vi "InitializeFpgaAcquisition.vi"(8 "error in (no error)":errorcluster, 11 "923x Acquisition Config":T1={"Acq"=FALSE, "NumberOfModules"=0, "Dynamic FPGA VI Ref"=refnum, "KeyphasorX3"=[], "FixedSizeX32"={"EnabledChannels"=[], "Sensitivity"=[], "InputConfig"=[]}, "SamplingInfo"={"Number of Channels"=4, "Sampling Rate"=4.0, "Channels"=[], "Units"=[], "Offsets"=[]}, "Normal Mode Sample Rate"=0.0, "BlockSize (sec)"=0.0, "Samples To Read (per chan)"=0, "RunningAcquisitionLength"=0.0, "Settling Time"=0.0, "Waveform Groups"=[], "Acquisition Block Number"=0, "Device Name"="", "ValidConfig"=FALSE, "Last Dynamic Module"="", "HighPassFilterState"=[], "Low Frequency Cutoff"=[], "BurstMode"={"Acquisition Time"=0.0, "Sample Rate"=0.0}} {"HighPassFilterState"."Filter State" format="%.2f"; "HighPassFilterState"."IIR Filter Cluster"."Forward Coefficients" format="%.2f"; "HighPassFilterState"."IIR Filter Cluster"."Reverse Coefficients" format="%.2f"; "FixedSizeX32"."InputConfig" items=["AC Coupled", "DC Coupled", "IEPE AC Coupled"]}) -> (0 "error out":errorcluster, 1 "start acquisition?":bool, 2 "dynamic FPGA VI reference":refnum<k20>, 3 "923x Acquisition Config out":T1={"Acq"=FALSE, "NumberOfModules"=0, "Dynamic FPGA VI Ref"=refnum, "KeyphasorX3"=[], "FixedSizeX32"={"EnabledChannels"=[], "Sensitivity"=[], "InputConfig"=[]}, "SamplingInfo"={"Number of Channels"=4, "Sampling Rate"=4.0, "Channels"=[], "Units"=[], "Offsets"=[]}, "Normal Mode Sample Rate"=0.0, "BlockSize (sec)"=0.0, "Samples To Read (per chan)"=0, "RunningAcquisitionLength"=0.0, "Settling Time"=0.0, "Waveform Groups"=[], "Acquisition Block Number"=0, "Device Name"="", "ValidConfig"=FALSE, "Last Dynamic Module"="", "HighPassFilterState"=[], "Low Frequency Cutoff"=[], "BurstMode"={"Acquisition Time"=0.0, "Sample Rate"=0.0}} {"HighPassFilterState"."Filter State" format="%.2f"; "HighPassFilterState"."IIR Filter Cluster"."Forward Coefficients" format="%.2f"; "HighPassFilterState"."IIR Filter Cluster"."Reverse Coefficients" format="%.2f"; "FixedSizeX32"."InputConfig" items=["AC Coupled", "DC Coupled", "IEPE AC Coupled"]})   [LabVIEW 2017, in "CmsAcquisition.lvlib"]
doc: "Initializes the acquisition of the dynamic channels with the RIO Wfm API."
uses:
  <vilib>/addons/InsightCM/Devices/Shared/Cms/CmsAcquisition/CmsAcquisition.lvlib
  <vilib>/addons/InsightCM/Devices/Shared/Cms/CmsAcquisition/controls/Configuration.ctl
  <vilib>/addons/InsightCM/Devices/Shared/Cms/CmsAcquisition/controls/TachometerConfig.ctl
  <vilib>/addons/InsightCM/Devices/Shared/Cms/CmsAcquisition/controls/FixedSizeArrays.ctl
  <vilib>/LabVIEW Targets/FPGA/cRIO/shared/nicrio_ModuleControls/nicrio_cRIO-9232_ConfigModeRing.ctl
  <vilib>/addons/InsightCM/Devices/Shared/Cms/cRIOWfmAcq/subVIs/RIO Wfm Cust Ctrls/rwfm_SamplingInfo.ctl
  <vilib>/addons/InsightCM/Devices/Shared/Cms/CmsAcquisition/controls/Group.ctl
  <vilib>/addons/InsightCM/Devices/Shared/Cms/CmsAcquisition/controls/Channel.ctl
  <vilib>/addons/InsightCM/Utilities/Analysis/Vibration/controls/HighPassFilterState.ctl
  <vilib>/addons/InsightCM/Devices/Shared/Cms/CmsAcquisition/controls/BurstMode.ctl
  <vilib>/Utility/error.llb/Error Cluster From Error Code.vi
  <vilib>/rvi/errors/niLvFpgaAdjustHostInterfaceError.vi
  <vilib>/rvi/interface/nirviReadWriteControl/nirviReadWriteControl.xnode
  <vilib>/addons/InsightCM/Devices/Shared/Cms/cRIOWfmAcq/cRIOWfmLib.lvlib
  NiFpgaLv.dll
  <vilib>/rvi/interface/Simulation/niFpgaSimulationCallBeginRW.vi
  <vilib>/addons/InsightCM/Utilities/Analysis/Vibration/VibrationAnalysisFunctions.lvlib
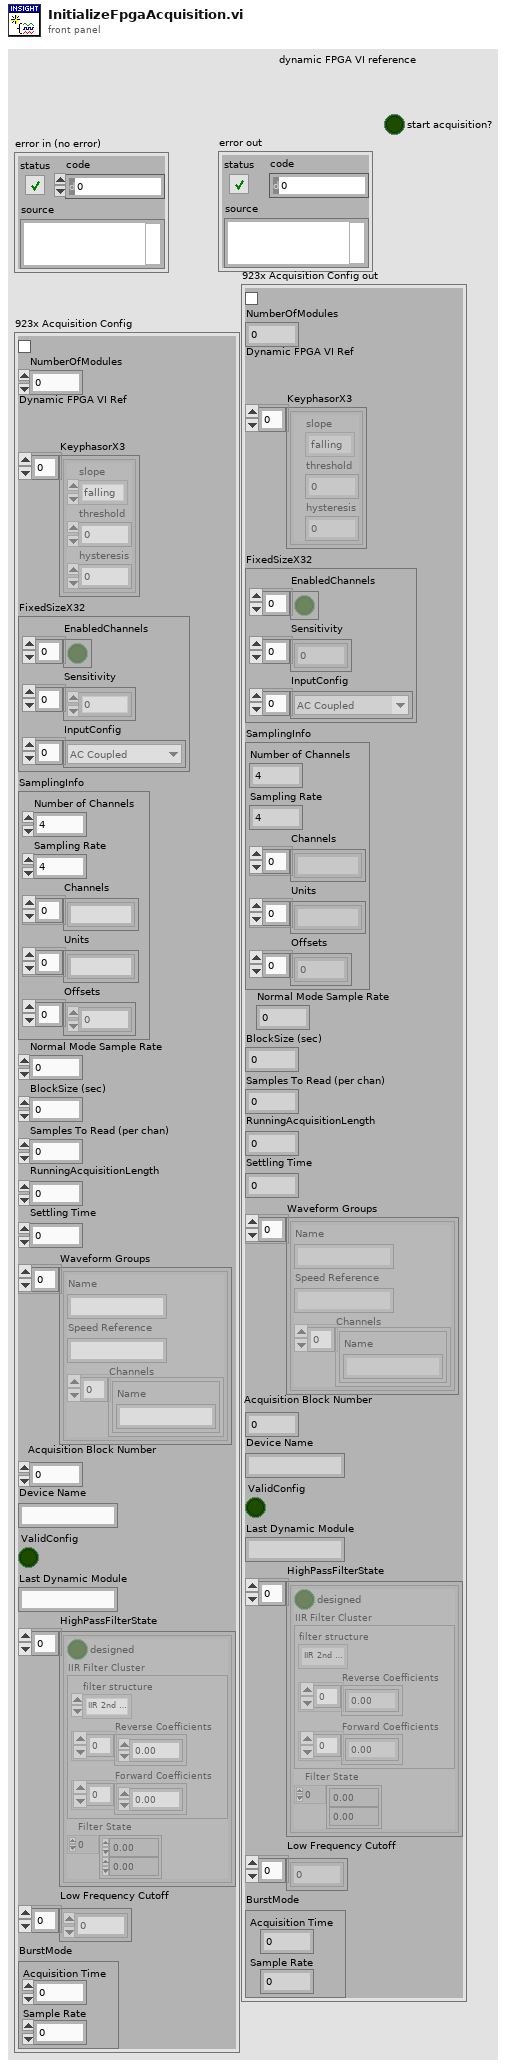
[diagram p1: front panel]
types:
  T1 = typedef "CmsAcquisition.lvlib/Configuration.ctl" = cluster{"Acq":bool, "NumberOfModules":i16, "Dynamic FPGA VI Ref":refnum<k20>, "KeyphasorX3":T2[], "FixedSizeX32":T3, "SamplingInfo":T5, "Normal Mode Sample Rate":dbl, "BlockSize (sec)":dbl, "Samples To Read (per chan)":i32, "RunningAcquisitionLength":dbl, "Settling Time":dbl, "Waveform Groups":T6[], "Acquisition Block Number":i32, "Device Name":string, "ValidConfig":bool, "Last Dynamic Module":string, "HighPassFilterState":T8[], "Low Frequency Cutoff":dbl[], "BurstMode":T9}
  T2 = typedef "CmsAcquisition.lvlib/TachometerConfig.ctl" = cluster{"slope":enum16{"falling", "rising"}, "threshold":dbl, "hysteresis":dbl}
  T3 = typedef "CmsAcquisition.lvlib/FixedSizeArrays.ctl" = cluster{"EnabledChannels":bool[], "Sensitivity":dbl[], "InputConfig":T4[]}
  T4 = typedef "nicrio_cRIO-9232_ConfigModeRing.ctl" = u8
  T5 = typedef "cRIOWfmLib.lvlib/rwfm_SamplingInfo.ctl" = cluster{"Number of Channels":i32, "Sampling Rate":dbl, "Channels":string[], "Units":string[], "Offsets":sgl[]}
  T6 = typedef "CmsAcquisition.lvlib/Group.ctl" = cluster{"Name":string, "Speed Reference":string, "Channels":T7[]}
  T7 = typedef "CmsAcquisition.lvlib/Channel.ctl" = cluster{"Name":string}
  T8 = typedef "VibrationAnalysisFunctions.lvlib/HighPassFilterState.ctl" = cluster{"designed":bool, "IIR Filter Cluster":cluster{"filter structure":enum32{"IIR 2nd Order", "IIR 4th Order"}, "Reverse Coefficients":dbl[], "Forward Coefficients":dbl[]}, "Filter State":dbl[]}
  T9 = typedef "CmsAcquisition.lvlib/BurstMode.ctl" = cluster{"Acquisition Time":dbl, "Sample Rate":dbl}
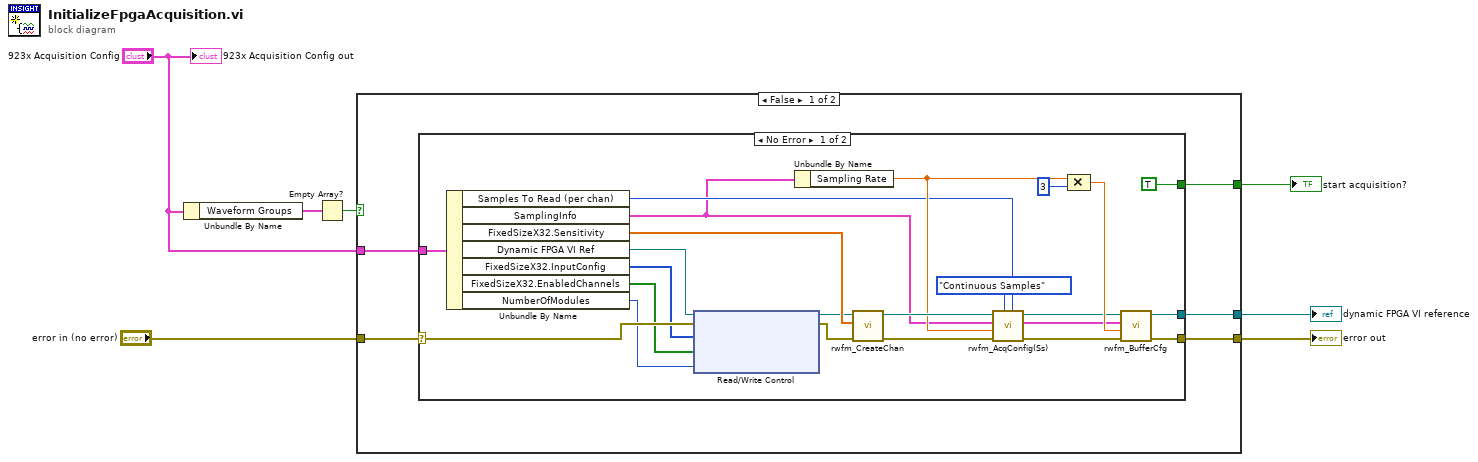
[diagram p0: block diagram]
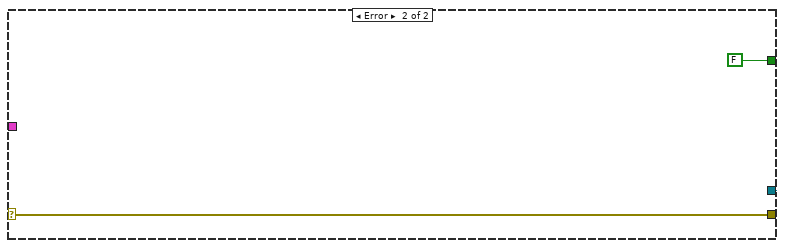
[diagram p2: hidden frame]
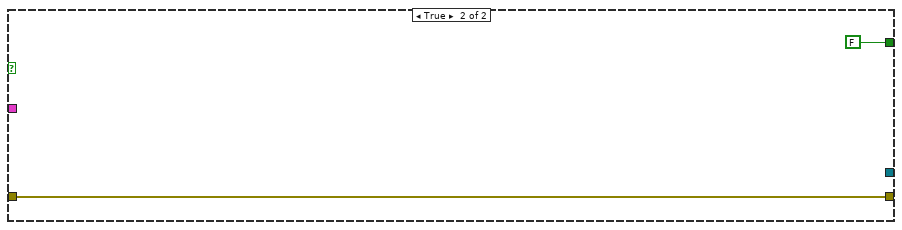
[diagram p3: hidden frame]
diagram:
  n1 = Unbundle By Name("923x Acquisition Config") -> ("Waveform Groups"=w4:T6[])
  n2 = Empty Array?(array=w4) -> (empty?=w2:bool)
  n3 = case shown="False" w2 {
    tunnel: "923x Acquisition Config" -> [w12 _]
    tunnel: [w11 w40] -> w7
    tunnel: "error in (no error)" -> [w10 w40]
    tunnel: [w9 _] -> w5
    tunnel: [w8 FALSE] -> w3
    frame False {
      n4 = case shown="No Error" w10 {
        selector: w10 -> [w31 w37]
        tunnel: w12 -> [w34 _]
        tunnel: [w33 w37] -> w11
        tunnel: [w32 refnum<k0> refnum] -> w9
        tunnel: [TRUE FALSE] -> w8
        frame No Error {
          n5 = Unbundle By Name(w34) -> ("Samples To Read (per chan)"=w18:i32, "SamplingInfo"=w14:T5, "FixedSizeX32.Sensitivity"=w35:dbl[], "Dynamic FPGA VI Ref"=w30:refnum<k20>, "FixedSizeX32.InputConfig"=w15:T4[], "FixedSizeX32.EnabledChannels"=w16:bool[], "NumberOfModules"=w17:i16)
          n6 = xnode "Read/Write Control"("FPGA VI Reference In"=w30, "error in"=w31, "Input Config Array"=w15, "Enable Chan Array"=w16, "Number of Modules"=w17) -> ("FPGA VI Reference Out"=w29:refnum<k20>, "error out"=w24:errorcluster)
          n7 = Unbundle By Name(w14) -> ("Sampling Rate"=w19:dbl)
          n8 = call <vilib>:"rwfm_CreateChan.vi"("error in"=w24, "Sensitivity"=w35, "Dynamic FPGA VI Reference"=w29) -> ("error out"=w20:errorcluster, "Dynamic FPGA VI Reference"=w21:refnum<k20>)  [unwired: 7 in]
          n9 = call <vilib>:"rwfm_AcqConfig(Ss).vi"("Samples per Channel"=w18, "Sample Mode"=enum16{"Finite Samples", "Continuous Samples"}."Continuous Samples", "error in"=w20, "Sample Rate S/s"=w19, "Sampling Info In"=w14, "Dynamic FPGA Ref"=w21) -> ("error out"=w22:errorcluster, "Sampling Info Out"=w26:T5, "Dynamic FPGA Ref Out"=w23:refnum<k20>)  [unwired: 2 in, 1 out]
          n10 = Compound Arithmetic op=MULTIPLY(w19, 3 ("value")) -> (w27:dbl)
          n11 = call <vilib>:"rwfm_BufferCfg.vi"("error in"=w22, "Buffer Size [Samps per Chan]"=w27, "Sampling Info In"=w26, "Dynamic FPGA VI Reference"=w23) -> ("error out"=w33:errorcluster, "Dynamic FPGA VI Reference"=w32:refnum<k20>)  [unwired: 4 in, 2 out]
        }
        frame Error {
          (unwired) cluster{"valid":bool, "description":string} {"valid"=FALSE, "description"=""} ("ConfigStatus")
        }
      }
    }
    frame True {
    }
  }
  "error out" <- w7
  "dynamic FPGA VI reference" <- w5
  "start acquisition?" <- w3
  "923x Acquisition Config out" <- "923x Acquisition Config"
